vi "GetLastRowExcel.vi"(8 "error in (no error)":errorcluster, 11 "report in":refnum<class "NI_report.lvclass">) -> (0 "error out":errorcluster, 2 "row":i32, 3 "report out":refnum<class "NI_report.lvclass">)   [LabVIEW 2012]
uses:
  <vilib>/Utility/NIReport.llb/NI_report.lvclass
  <vilib>/Utility/NIReport.llb/Excel/NI_Excel.lvclass
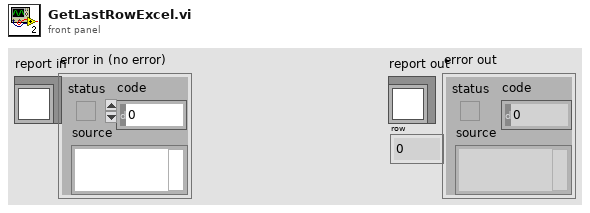
[diagram p1: front panel]
types:
  T1 = cluster{"position (Excel)":cluster{"row":i32, "column":i32}, "name (Excel)":string, "bookmark (Word)":string}
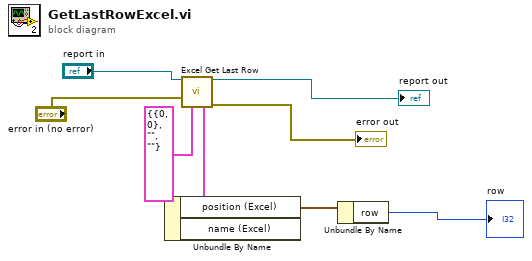
[diagram p0: block diagram]
diagram:
  n1 = call <vilib>:"Excel Get Last Row.vi"("report in"="report in", "error in (no error)"="error in (no error)", "MS Office parameters"=T1 {"position (Excel)"={"row"=0, "column"=0}, "name (Excel)"="", "bookmark (Word)"=""}) -> ("report out"=→"report out":refnum<class "NI_report.lvclass">, "MS Office parameters out"=w3:T1, "error out"=→"error out":errorcluster)  [unwired: 10 in]
  n2 = Unbundle By Name(w3) -> ("position (Excel)"=w1:cluster{"row":i32, "column":i32})  [unwired: 1 out]
  n3 = Unbundle By Name(w1) -> ("row"=→"row":i32)
